vi "Write_control_mode.vi"(11 "Control_Mode":T1(ring)) -> ()   [LabVIEW 2014]
uses:
  ctl/P3AT_Current.ctl
  Global_var.vi
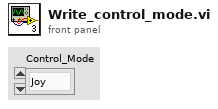
[diagram p1: front panel]
types:
  T1 = enum32{"Joy", "Map", "Voice", "Input", "Undefined"}
  T2 = typedef "P3AT_Current.ctl" = cluster{"max_vel":dbl, "max_rot":dbl, "now_pose_X":dbl, "now_pose_Y":dbl, "now_pose_Rot_deg":dbl, "Control_Mode":enum32{"Joy", "Map", "Voice", "Input", "Undefined"}}
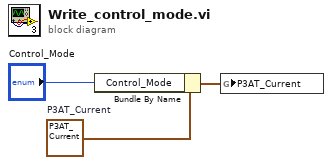
[diagram p0: block diagram]
diagram:
  w3 = T2 {"max_vel"=0.49056603773584906, "max_rot"=0.5094339622641509, "now_pose_X"=0.0, "now_pose_Y"=0.0, "now_pose_Rot_deg"=0.0, "Control_Mode"=enum."Joy"}  # P3AT_Current
  n1 = Bundle By Name(cluster=w3, "Control_Mode"="Control_Mode") -> (w2:T2)
  n2 = global write "Global_var.vi" "P3AT_Current"(w2) -> ()
